vi "_Convert Virtual Channel.vi"(2 "DAC":u32, 3 "Ch#":u8) -> (0 "DAC Out":u32, 1 "Ch# Out":u8)   [LabVIEW 2015]
uses:
  Type/_FPGA Chip Type.ctl
  <vilib>/rvi/Memory/Memory_Emulation/nirvimemoryFastEmulation.vi
  <vilib>/rvi/Memory/Memory_Emulation/nirvimemoryEmulation.vi
  <vilib>/rvi/Emulation/niFpgaEmulationIsFPGAContextNoSignature.vi
  <vilib>/rvi/DataTransferAndStorage/Container/Common/niFpgaContainerGetUniqueNameForEmu.vi
  <vilib>/rvi/Emulation/niFpgaProcessEmulError.vi
  <vilib>/rvi/Emulation/niFpgaSctlEmulationGetInTimedLoop.vi
  <vilib>/rvi/errors/nirviReportUnexpectedCaseInternalError (U32).vi
  <vilib>/rvi/eio/common/nirviEmuTemplateMethod_errors.vi
  <vilib>/rvi/DataTransferAndStorage/Container/XNode/niFpgaContainer.xnode
  <vilib>/eio/EIONode/EIONode.xnode
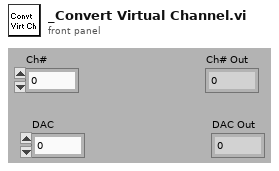
[diagram p1: front panel]
types:
  T1 = typedef "_FPGA Chip Type.ctl" = enum8{"None", "ADC1", "ADC2", "ADC3", "ADC4", "ADC5", "ADC6", "ADC7", "ADC8", "ADC9", "ADC10", "ADC11", "ADC12", "ADC13", "DAC1", "DAC2", "DAC3", "DAC4", "DAC5", "LENS1", "LENS2", "LENS3", "LENS4", "LENS5", "LENS6", "LENS7", "MASS1", "MASS2", "MASS3", "MASS4", "MASS5", "OSC1", "OSC2", "OSC3", "LATCH1", "LATCH2", "LATCH3", "LATCH4", "PIC1", "PIC2", "PIC3", "PIC4"}
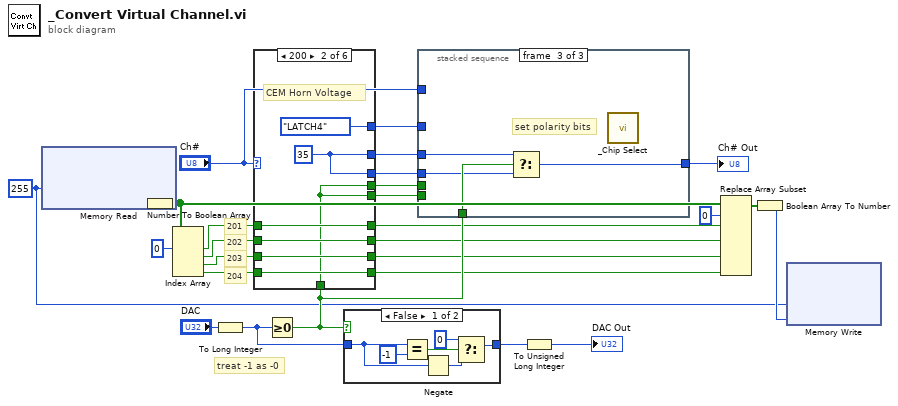
[diagram p0: block diagram]
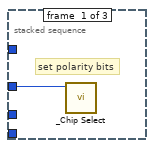
[diagram p3: hidden frame]
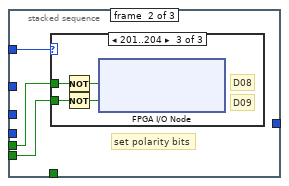
[diagram p4: hidden frame]
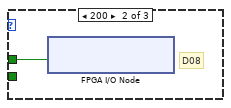
[diagram p6: hidden frame]
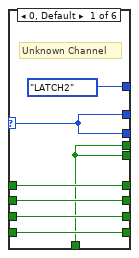
[diagram p7: hidden frame]
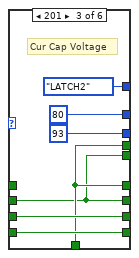
[diagram p8: hidden frame]
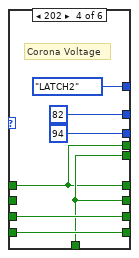
[diagram p9: hidden frame]
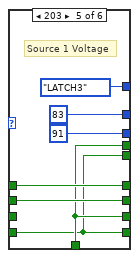
[diagram p10: hidden frame]
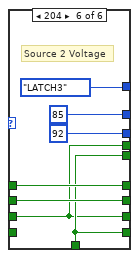
[diagram p11: hidden frame]
diagram:
  w1 = u32 255 ("Address")
  # "treat -1 as -0"
  # "204"
  # "203"
  # "202"
  # "201"
  n1 = xnode ("Memory Read")("Address"=w1) -> ("Data"=w27:u32)  [unwired: 1 in, 1 out]
  n2 = Number To Boolean Array(number=w27) -> (Boolean array=w7:bool[])
  n3 = Index Array(array=w7, index #1=0 ("index")) -> (element #1=w13:bool, element #2=w12:bool, element #3=w11:bool, element #4=w10:bool)  [unwired: 3 in]
  n4 = To Long Integer(number="DAC") -> (32bit integer=w16:i32)
  n5 = Greater Or Equal To 0?(x=w16) -> (x >= 0?=w15:bool)
  n6 = case shown="200" "Ch#" {
    selector: "Ch#" -> [w34 _ _ _ _ _]
    tunnel: [w34 w40 u8 80 ("y") u8 82 ("y") u8 83 ("y") u8 85 ("y")] -> w20
    tunnel: [w34 w40 u8 93 ("y") u8 94 ("y") u8 91 ("y") u8 92 ("y")] -> w19
    tunnel: [_FPGA_Chip_Type."LATCH2" ("ChipType") _FPGA_Chip_Type."LATCH4" ("ChipType") _FPGA_Chip_Type."LATCH2" ("ChipType") _FPGA_Chip_Type."LATCH2" ("ChipType") _FPGA_Chip_Type."LATCH3" ("ChipType") _FPGA_Chip_Type."LATCH3" ("ChipType")] -> w21
    tunnel: w15 -> [w28 w35 w43 w50 w57 w64]
    tunnel: [w32 w36 w43 w49 w58 w65] -> w3
    tunnel: [w31 w39 w42 w50 w59 w66] -> w4
    tunnel: [w30 w38 w45 w52 w57 w63] -> w5
    tunnel: [w29 w37 w44 w51 w56 w64] -> w6
    tunnel: w12 -> [w31 w39 w42 _ w59 w66]
    tunnel: w11 -> [w30 w38 w45 w52 _ w63]
    tunnel: w10 -> [w29 w37 w44 w51 w56 _]
    tunnel: w13 -> [w32 w36 _ w49 w58 w65]
    tunnel: [w28 w35 w43 w49 w57 w63] -> w18
    tunnel: [w28 w35 w42 w50 w56 w64] -> w17
    frame 0, Default {
      # "Unknown Channel"
    }
    frame 200 {
      w40 = u8 35 ("y")
      # "CEM Horn Voltage"
    }
    frame 201 {
      # "Cur Cap Voltage"
    }
    frame 202 {
      # "Corona Voltage"
    }
    frame 203 {
      # "Source 1 Voltage"
    }
    frame 204 {
      # "Source 2 Voltage"
    }
  }
  n7 = case shown="False" w15 {
    tunnel: [w74 w76] -> w14
    tunnel: w16 -> [w71 w76]
    frame False {
      n8 = Equal?(x=w71, y=-1) -> (x = y?=w73:bool)
      n9 = Negate(x=w71) -> (-x=w70:i32)
      n10 = Select(t=0 ("y"), s=w73, f=w70) -> (s? t:f=w74:i32)
    }
    frame True {
    }
  }
  n11 = stacked-sequence {
    tunnel: w21 -> [w77 _ _]
    tunnel: w15 -> [_ _ w89]
    tunnel: "Ch#" -> [_ w80 _]
    tunnel: w20 -> [_ _ w88]
    tunnel: w19 -> [_ _ w87]
    tunnel: [_ _ w86] -> w24
    tunnel: w18 -> [_ w79 _]
    tunnel: w17 -> [_ w78 _]
    frame #0 {
      # "set polarity bits"
      n12 = call "_Chip Select.vi"("ChipType"=w77) -> ()  [unwired: 1 in, 6 out]
    }
    frame #1 {
      # "set polarity bits"
      n13 = case shown="201..204" w80 {
        tunnel: w79 -> [_ w81 w85]
        tunnel: w78 -> [_ _ w84]
        frame 0, Default {
        }
        frame 200 {
          # "D08"
          n14 = xnode "FPGA I/O Node"("Digtal IO/DIO34"=w81) -> ()  [unwired: 1 in, 1 out]
        }
        frame 201..204 {
          # "D09"
          # "D08"
          n15 = Not(x=w85) -> (.not. x?=w83:bool)
          n16 = Not(x=w84) -> (.not. x?=w82:bool)
          n17 = xnode "FPGA I/O Node"("Digtal IO/DIO34"=w83, "Digtal IO/DIO32"=w82) -> ()  [unwired: 2 in, 2 out]
        }
      }
    }
    frame #2 {
      # "set polarity bits"
      n18 = Select(t=w88, s=w89, f=w87) -> (s? t:f=w86:u8)
      n19 = call "_Chip Select.vi"() -> ()  [unwired: 2 in, 6 out]
    }
  }
  "Ch# Out" <- w24
  n20 = To Unsigned Long Integer(number=w14) -> (unsigned 32bit integer=→"DAC Out":u32)
  n21 = Replace Array Subset(array=w7, new element #1=w3, index #1=0 ("index"), new element #2=w4, new element #3=w5, new element #4=w6) -> (w8:bool[])  [unwired: 3 in]
  n22 = Boolean Array To Number(Boolean array=w8) -> (number=w2:u32)
  n23 = xnode ("Memory Write")("Address"=w1, "Data"=w2) -> ()  [unwired: 1 in, 1 out]
